vi "test_fpga_rmp_main.vi"() -> ()   [LabVIEW 2016]
uses:
  <vilib>/Platform/TimedLoop/XDataNode/timing_clust.ctl
  <vilib>/Platform/TimedLoop/XDataNode/nitl_modes.ctl
  <vilib>/Platform/TimedLoop/XDataNode/wakeup.ctl
  <vilib>/rvi/Emulation/niFpgaSctlEmulationGetInTimedLoop.vi
  <vilib>/rvi/Emulation/niFpgaEmulationReportErrorSimple.vi
  <vilib>/rvi/Emulation/niFpgaGetClockAttributes.vi
  <vilib>/rvi/Emulation/niFpgaCriticalErrorInLSC.vi
  <vilib>/Platform/TimedLoop/XDataNode/XDataNode.xnode
  <vilib>/Platform/TimedLoop/XDataNode/XDNodeRunTimeDep.lvlib
panel:
  in  "rmp.p.simIn":T1 {"rmp.p.procVar" format="%#_13g"}
  out "rmp.o.height":T2
  out "rmp.o.debug":cluster{"rmp.s.running":bool}
  in  "rmp.p.params":T3
  in  "rmp.p.triggerParams":T4 {"rmp.triggerSource" items=["Absolute z height", "Process variable", "External"]}
  in  "rmp.p.start":bool
  in  "rmp.p.resetStartPos":bool
  in  "rmp.i.externalTrigger":bool
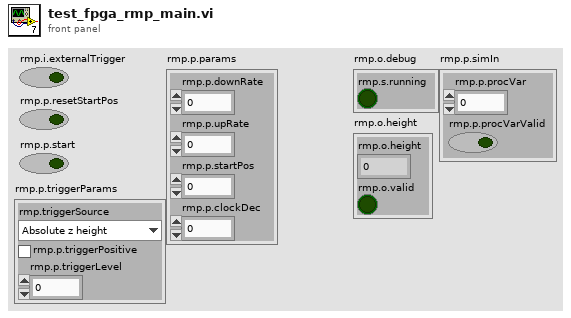
[diagram p1: front panel]
types:
  T1 = cluster{"rmp.p.procVar":fxp<+/-,24,16>, "rmp.p.procVarValid":bool}
  T2 = cluster{"rmp.o.height":fxp<+/-,24,2>, "rmp.o.valid":bool}
  T3 = cluster{"rmp.p.downRate":fxp<+/-,22,1>, "rmp.p.upRate":fxp<+/-,22,1>, "rmp.p.startPos":fxp<+/-,24,2>, "rmp.p.clockDec":u16}
  T4 = cluster{"rmp.triggerSource":u8, "rmp.p.triggerPositive":bool, "rmp.p.triggerLevel":fxp<+/-,24,16>}
  T5 = typedef "XDNodeRunTimeDep.lvlib/timing_clust.ctl" = cluster{"Expected End [f-1]":u64, "Actual End [f-1]":u64, "Finished Late? [f-1]":bool, "Expected End [i-1]":u64, "Actual End [i-1]":u64, "Finished Late? [i-1]":bool, "Expected Start [i]":u64, "Actual Start [i]":u64, "Expected Start [f]":u64, "Actual Start [f]":u64, "Source Name":string, "Structure Name":string, "Period":i64, "Deadline":i64, "Offset":i64, "Start":i64, "Priority":i32, "Timeout":i32, "Mode":T6, "Wakeup Reason":T7, "Error":errorcluster, "Source Type":string, "Secondary Source Type":string, "Global End Time":u64, "Global Start Time":u64, "Frame Duration":u64, "Iteration Duration":u64, "Assigned CPU":i32, "I/O Scan Engine Mode":u32}
  T6 = typedef "XDNodeRunTimeDep.lvlib/nitl_modes.ctl" = enum32{"No Change", "Process missed periods, maintain original phase", "Discard missed periods, maintain original phase", "Process missed periods, ignore original phase", "Discard missed periods, ignore original phase"}
  T7 = typedef "XDNodeRunTimeDep.lvlib/wakeup.ctl" = enum32{"Normal", "Aborted", "Asynchronous wakeup", "Timing source error", "Timed loop error", "Timeout"}
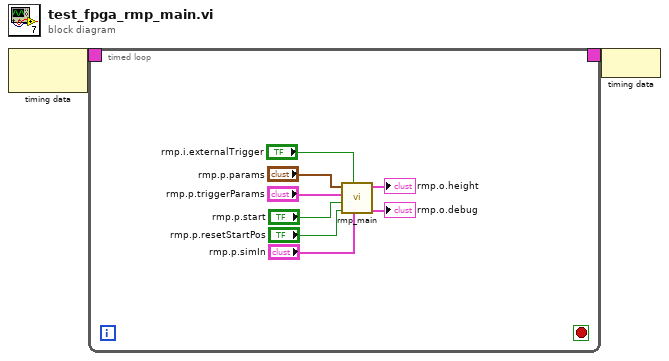
[diagram p0: block diagram]
diagram:
  n1 = node-c288() -> (w2:T5)  [unwired: 1 in]
  n2 = timed-loop {
    timing: w2 -> [_]
    timing-out: [_] -> w1
    stop <- _ stop-if-true
    n3 = call "rmp_main.vi"("rmp.p.simIn"="rmp.p.simIn", "rmp.i.externalTrigger"="rmp.i.externalTrigger", "rmp.p.resetStartPos"="rmp.p.resetStartPos", "rmp.p.start"="rmp.p.start", "rmp.p.triggerParams"="rmp.p.triggerParams", "rmp.p.params"="rmp.p.params") -> ("rmp.o.debug"=→"rmp.o.debug":cluster{"rmp.s.running":bool}, "rmp.o.height"=→"rmp.o.height":T2)  [unwired: 4 in]
  }
  n4 = node-c288(w1) -> ()
